vi "Control Init.vi"(7 "VolatusAPI":refnum<class "VolatusAPI.lvclass">, 8 "error in (no error)":errorcluster, 10 "JSON":string, 11 "DblPopupControl in":refnum<class "DblPopupControl.lvclass">) -> (0 "error out":errorcluster, 3 "DblPopupControl out":refnum<class "DblPopupControl.lvclass">)   [LabVIEW 2020, in "VolatusGUIElements.lvlib" / "DblPopupControl.lvclass"]
uses:
  DblPopupControl.lvclass
  C:/dev/lv20CE/relink/lv-volatus/VolatusGUI/GUI Element/GUI Element.lvclass
  Volatus/VolatusAPI/VolatusAPI.lvclass
  JSON.ctl
  Cmd State.ctl
  VolatusGUI/GUI Element/GUI Element.lvclass/GUI Element.ctl
  DblPopupControl.lvclass/DblPopupControl.ctl
  9743c59a-7e7e-4945-bb31-9bc961dfa8ed.vi
  <vilib>/JDP Science/JSONtext/JSON text to Variant.vi
  <vilib>/JDP Science/JSONtext/LVClass Serializer/JSONtext LVClass Serializer.lvclass
  VolatusGUI/GUI Element/GUI Element.lvclass
  VolatusGUIElements.lvlib
  lv-vecto/Vecto/Group/Group.lvclass
  C:/dev/lv20CE/relink/lv-vecto/Vecto/GroupAbstract/GroupAbstract.lvclass
  C:/dev/lv20CE/relink/lv-vecto/Vecto/Group/Group.lvclass
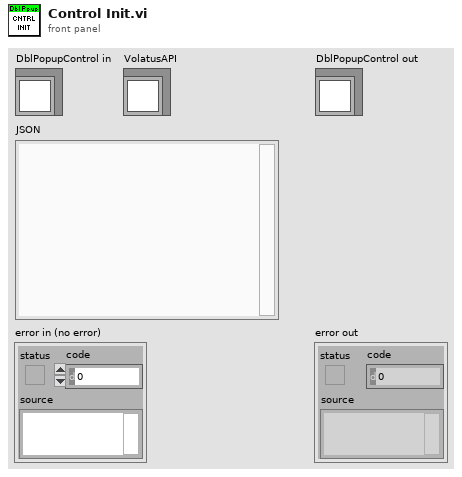
[diagram p1: front panel]
types:
  T1 = typedef "VolatusGUIElements.lvlib/DblPopupControl.lvclass/Cmd State.ctl" = cluster{"Commanding":bool, "Start":dbl, "Error":bool, "Value":dbl}
  T2 = typedef "VolatusGUIElements.lvlib/DblPopupControl.lvclass/JSON.ctl" = cluster{"Channel":string, "Format":string, "Color":cluster{"Text":string, "BG":string}, "Staleness":dbl}
  T3 = typedef "VectoConfig.lvlib/Channel Info.ctl" = cluster{"Name":string, "Group":string, "Owning Node":string, "Owning Task":string, "Resource":string}
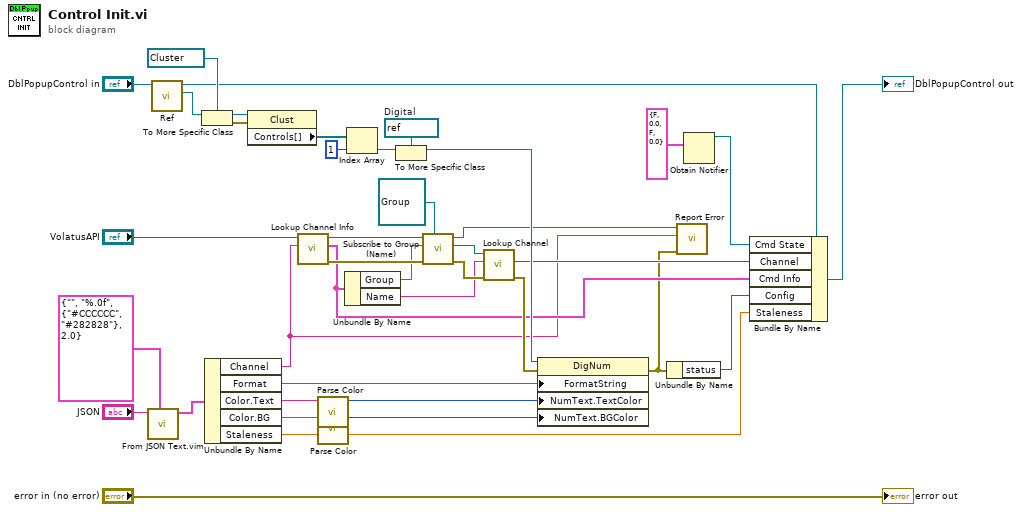
[diagram p0: block diagram]
diagram:
  w30 = refnum<vi> refnum  # Digital
  n1 = call "From JSON Text.vim"("Data Type and Default Value"=T2 {"Channel"="", "Format"="%.0f", "Color"={"Text"="#CCCCCC", "BG"="#282828"}, "Staleness"=2.0} ("JSON"), "JSON"="JSON") -> ("Data out"=w35:T2)  [unwired: 8 in, 1 out]
  n2 = call "Ref.vi"("GUI Element in"="DblPopupControl in") -> ("Ref"=w34:refnum<vi>, "GUI Element out"=w11:refnum<class "DblPopupControl.lvclass">)  [unwired: 9 in]
  n3 = To More Specific Class(target class=refnum<vi> refnum ("specific class reference"), reference=w34) -> (specific class reference=w32:refnum<vi>, error out=w31:errorcluster)  [unwired: 1 in]
  n4 = Unbundle By Name(w35) -> ("Channel"=w1:string, "Format"=w22:string, "Color.Text"=w24:string, "Color.BG"=w23:string, "Staleness"=w7:dbl)
  n5 = property class="Clust"(reference=w32, error in=w31) -> ("Controls[]"=w29:refnum<vi>[])  [unwired: 2 out]
  n6 = call "Lookup Channel Info.vi"("Channel Name"=w1, "VolatusAPI in"="VolatusAPI") -> ("error out"=w16:errorcluster, "Channel Info"=w9:T3, "VolatusAPI out"=w15:refnum<class "VolatusAPI.lvclass">)  [unwired: 6 in, 1 out]
  n7 = call "Parse Color.vi"("Color String"=w24) -> ("Color"=w21:u32)  [unwired: 9 in, 1 out]
  n8 = call "Parse Color.vi"("Color String"=w23) -> ("Color"=w20:u32)  [unwired: 9 in, 1 out]
  n9 = Unbundle By Name(w9) -> ("Group"=w14:string, "Name"=w13:string)
  n10 = Index Array(array=w29, index=1) -> (element=w27:refnum<vi>)
  n11 = To More Specific Class(target class=w30, reference=w27) -> (specific class reference=w25:refnum<vi>)  [unwired: 1 in, 1 out]
  n12 = call "Subscribe to Group (Name).vi"("Group Type"=refnum<class "Group.lvclass"> refnum ("Vecto.lvlib:Group.lvclass"), "error in (no error)"=w16, "Group Name"=w14, "VolatusAPI in"=w15) -> ("error out"=w17:errorcluster, "Group"=w18:refnum<class "Group.lvclass">, "VolatusAPI out"=w3:refnum<class "VolatusAPI.lvclass">)  [unwired: 5 in]
  n13 = call "Lookup Channel.vi"("error in (no error)"=w17, "Channel Name"=w13, "Group in"=w18) -> ("error out"=w39:errorcluster, "Channel"=w10:refnum<class "Channel.lvclass">)  [unwired: 6 in, 1 out]
  n14 = property class="DigNum"(reference=w25, error in=w39, "FormatString"=w22, "NumText.TextColor"=w21, "NumText.BGColor"=w20) -> (error out=w2:errorcluster)  [unwired: 1 out]
  n15 = Unbundle By Name(w2) -> ("status"=w8:bool)
  n16 = call "Report Error.vi"("error in (no error)"=w2, "Context"=w1, "VolatusAPI in"=w3) -> ()  [unwired: 7 in, 2 out]
  n17 = Obtain Notifier(notification data type=T1 {"Commanding"=FALSE, "Start"=0.0, "Error"=FALSE, "Value"=0.0} ("Cmd State")) -> (notifier out=w4:refnum<notifier>)  [unwired: 3 in, 2 out]
  n18 = Bundle By Name(cluster=w11, "Cmd State"=w4, "Channel"=w10, "Cmd Info"=w9, "Config"=w8, "Staleness"=w7) -> (→"DblPopupControl out":refnum<class "DblPopupControl.lvclass">)
  "error out" <- "error in (no error)"
